vi "Select display mode.vi"(8 "error in (no error)":errorcluster, 10 "Display":T1, 11 "VISA resource name":refnum<visa-resource-name>="GPIB0::21::INSTR") -> (0 "error out":errorcluster, 3 "VISA resource name out":refnum<visa-resource-name>)   [LabVIEW 2017, in "Anritsu Power Meter.lvlib"]
uses:
  Anritsu Power Meter.lvlib
  Display control.ctl
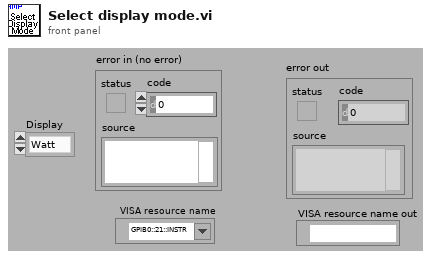
[diagram p1: front panel]
types:
  T1 = typedef "Anritsu Power Meter.lvlib/Display control.ctl" = enum16{"Watt", "dBm", "dB (REL)"}
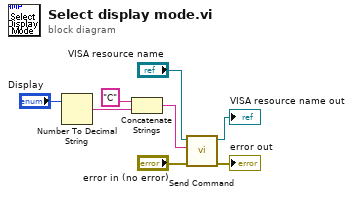
[diagram p0: block diagram]
diagram:
  n1 = Number To Decimal String(number="Display") -> (decimal integer string=w4:string)  [unwired: 1 in]
  n2 = Concatenate Strings("C" ("string"), w4) -> (w2:string)
  n3 = call "Send Command.vi"("error in (no error)"="error in (no error)", "write buffer"=w2, "VISA resource name"="VISA resource name") -> ("error out"=→"error out":errorcluster, "VISA resource name out"=→"VISA resource name out":refnum<visa-resource-name>)  [unwired: 7 in]
